vi "Send Mixed Mode Command.vi"(1 "MCL Command In":refnum<queue>, 2 "Ramp Times":cluster{"Displacement":T1, "Force":T1}, 3 "error in":errorcluster, 4 "Combined":bool) -> (5 "MCL Command Out":refnum<queue>, 6 "error out":errorcluster)   [LabVIEW 2013]
uses:
  Ramp Time Tuple.ctl
  Mixed Mode Command.ctl
  Mixed Mode Command Action.ctl
  Target Data.ctl
  Apps/On Off Button.ctl
  Data Access Objects/Metadata/DAO Actions.ctl
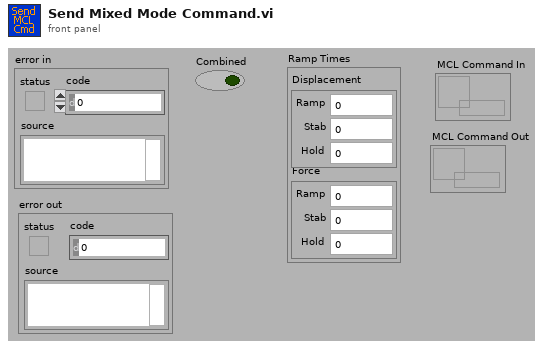
[diagram p1: front panel]
types:
  T1 = typedef "Ramp Time Tuple.ctl" = cluster{"Ramp":dbl, "Stab":dbl, "Hold":dbl}
  T2 = typedef "DAO Actions.ctl" = enum16{"Init", "Get", "Set"}
  T3 = typedef "On Off Button.ctl" = bool
  T4 = typedef "Mixed Mode Command.ctl" = cluster{"Command":T5, "Ramp Times":cluster{"Initial":T1, "Iterative":T1}, "LBCB1":T6, "LBCB2":T6}
  T5 = typedef "Mixed Mode Command Action.ctl" = enum16{"Start Command", "Stop", "Exit", "No Op", "Start Acquisition", "Measure Initial Position"}
  T6 = typedef "Target Data.ctl" = cluster{"Displacements":dbl[], "Command Type":enum16{"<None>", "Displacement", "Force"}[], "Forces":dbl[]}
  T7 = typedef "Target.ctl" = cluster{"LBCB Number":T8, "DOF Vectors":enum16{" ", "Dx", "Dy", "Dz", "Rx", "Ry", "Rz", "Fx", "Fy", "Fz", "Mx", "My", "Mz"}, "Amount":dbl}
  T8 = typedef "LBCB Number.ctl" = enum16{"LBCB1", "LBCB2"}
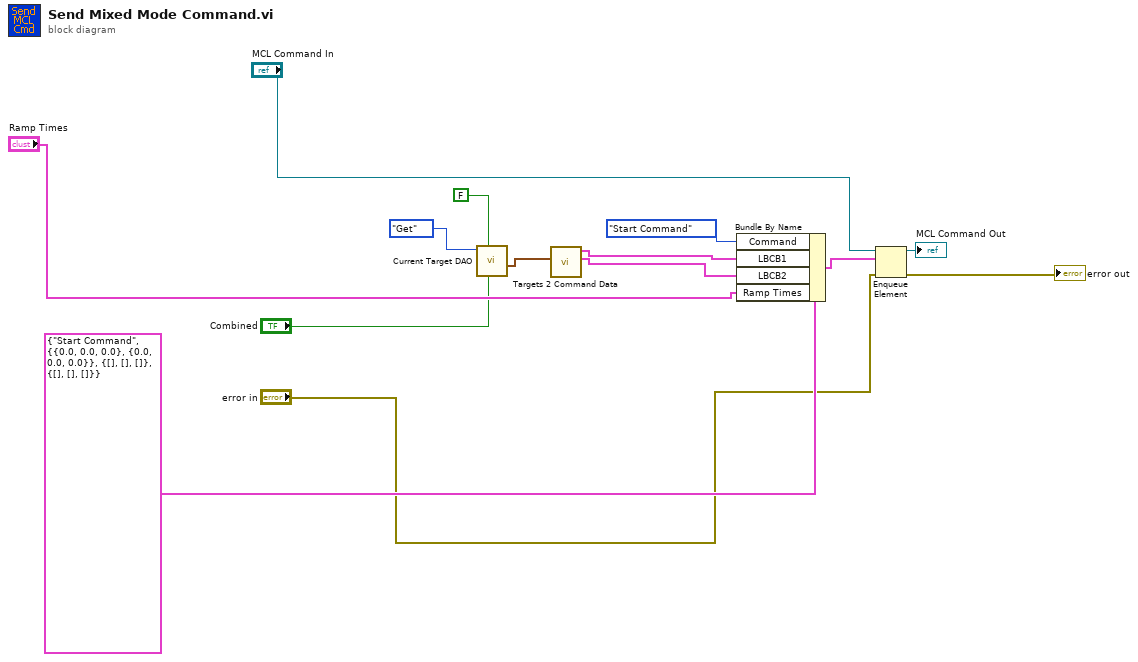
[diagram p0: block diagram]
diagram:
  n1 = call "Current Target DAO.vi"("Combined"="Combined", "Use Offsets"=T3 FALSE, "DAO Actions"=DAO_Actions."Get") -> ("Targets  Out"=w5:T7[])  [unwired: 7 in, 1 out]
  n2 = call "Targets 2 Command Data.vi"("Target  Inputs"=w5) -> ("LBCB 2 Command Data"=w8:T6, "LBCB 1 Command Data"=w7:T6)  [unwired: 1 in, 8 out]
  n3 = Bundle By Name(cluster=T4 {"Command"=enum."Start Command", "Ramp Times"={"Initial"={"Ramp"=0.0, "Stab"=0.0, "Hold"=0.0}, "Iterative"={"Ramp"=0.0, "Stab"=0.0, "Hold"=0.0}}, "LBCB1"={"Displacements"=[], "Command Type"=[], "Forces"=[]}, "LBCB2"={"Displacements"=[], "Command Type"=[], "Forces"=[]}} ("Mixed Mode Command In"), "Command"=Mixed_Mode_Command_Action."Start Command", "LBCB1"=w7, "LBCB2"=w8, "Ramp Times"="Ramp Times") -> (w9:T4)
  n4 = Enqueue Element(queue="MCL Command In", element=w9, error in (no error)="error in") -> (queue out=→"MCL Command Out":refnum<queue>, error out=→"error out":errorcluster)  [unwired: 1 in, 1 out]
